vi "Get Vibration Profile.vi"(8 "error in (no error)":errorcluster, 11 "Config Data":T2) -> (0 "error out":errorcluster, 3 "Active Vibration Profile":T1)   [LabVIEW 2026, in "Acquisition.lvlib"]
uses:
  Acquisition.lvlib
  Controls/Vibration_Profile.ctl
  Controls/Vibration_Monitor_Config.ctl
  Controls/Options.ctl
  Controls/System_Settings.ctl
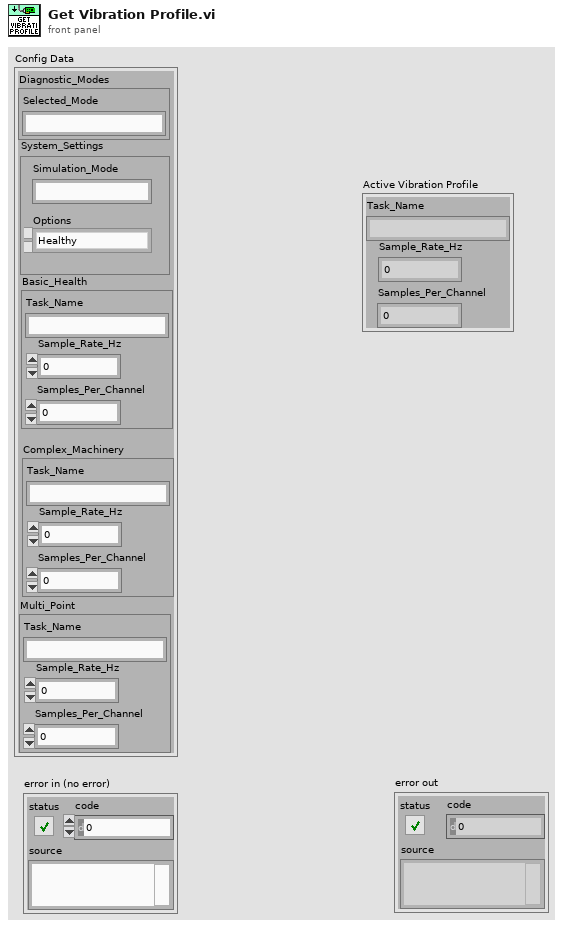
[diagram p1: front panel]
types:
  T1 = typedef "Vibration_Profile.ctl" = cluster{"Task_Name":string, "Sample_Rate_Hz":dbl, "Samples_Per_Channel":i32}
  T2 = typedef "Vibration_Monitor_Config.ctl" = cluster{"Diagnostic_Modes":cluster{"Selected_Mode":string}, "Basic_Health":T1, "Complex_Machinery":T1, "Multi_Point":T1, "System_Settings":T3}
  T3 = typedef "System_Settings.ctl" = cluster{"Simulation_Mode ":string, "Options":T4}
  T4 = typedef "Options.ctl" = enum16{"Healthy", "Unbalance_Alert", "Bearing_Fault_Critical", "Sweep_Test"}
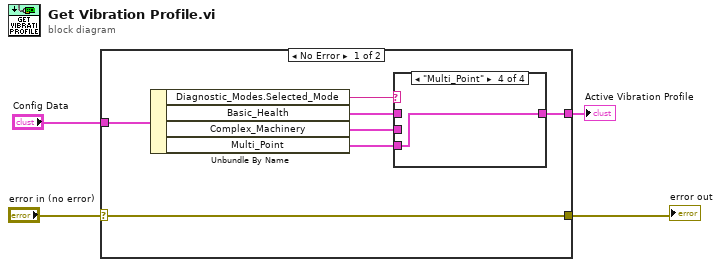
[diagram p0: block diagram]
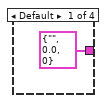
[diagram p2: hidden frame]
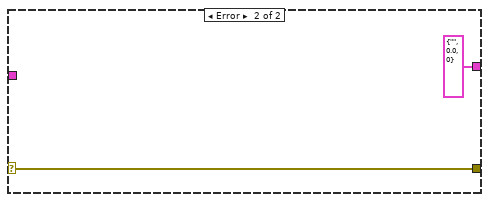
[diagram p5: hidden frame]
diagram:
  n1 = case shown="No Error" "error in (no error)" {
    selector: "error in (no error)" -> [w7 w17]
    tunnel: [w7 w17] -> w3
    tunnel: "Config Data" -> [w6 _]
    tunnel: [w5 T1 {"Task_Name"="", "Sample_Rate_Hz"=0.0, "Samples_Per_Channel"=0} ("Multi_Point")] -> w1
    frame No Error {
      n2 = Unbundle By Name(w6) -> ("Diagnostic_Modes.Selected_Mode"=w8:string, "Basic_Health"=w9:T1, "Complex_Machinery"=w10:T1, "Multi_Point"=w11:T1)
      n3 = case shown="\"Multi_Point\"" w8 {
        tunnel: [T1 {"Task_Name"="", "Sample_Rate_Hz"=0.0, "Samples_Per_Channel"=0} ("Multi_Point") w13 w14 w15] -> w5
        tunnel: w9 -> [_ _ w14 _]
        tunnel: w10 -> [_ w13 _ _]
        tunnel: w11 -> [_ _ _ w15]
        frame Default {
        }
        frame "Complex_Machinery" {
        }
        frame "Basic_Health" {
        }
        frame "Multi_Point" {
        }
      }
    }
    frame Error {
    }
  }
  "error out" <- w3
  "Active Vibration Profile" <- w1
